vi "DAQmx devices info.vi"() -> (0 "ArrayInfo":string[][](array[string]))   [LabVIEW 2018]
doc: "Ricava, in <B>ArrayInfo</B>, informazioni sui dispositivi installati"
uses:
  <resource>/objmgr/daqmx.rc
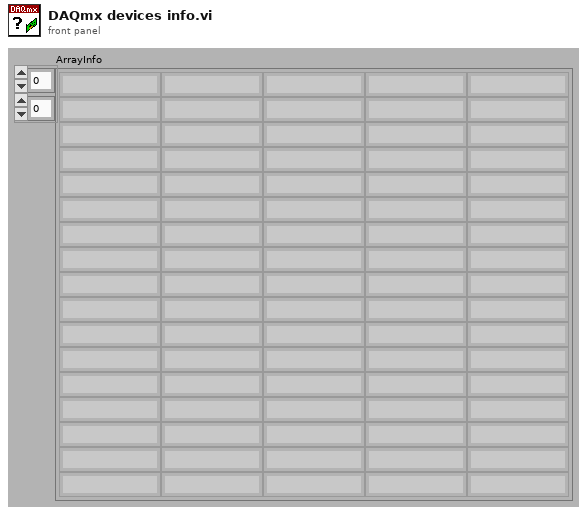
[diagram p1: front panel]
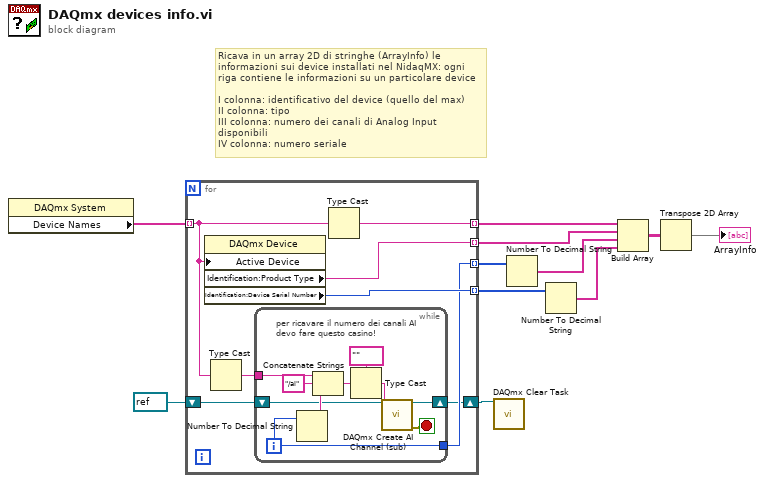
[diagram p0: block diagram]
diagram:
  # "Ricava in un array 2D di stringhe (ArrayInfo) le informazioni sui device installati nel NidaqMX: ogni riga contiene le informazioni su un particolare device\n\nI colonna: identificativo del device (quello del max)\nII colonna: tipo\nIII colonna: numero dei canali di Analog Input disponibili\nIV colonna: numero seriale"
  n1 = property class="DAQmx System"() -> ("Device Names"=w11:tag[])  [unwired: 2 in, 2 out]
  n2 = for {
    tunnel: w11 -> [w15] mode=indexing
    tunnel: [w19] -> w7 mode=indexing
    tunnel: [w18] -> w10 mode=indexing
    tunnel: [w16] -> w9 mode=indexing
    tunnel: [w14] -> w8 mode=indexing
    shift-right: [w13] -> w2
    shift-left: refnum<k21> refnum ("task in") -> [w12]
    n3 = property class="DAQmx Device"("Active Device"=w15) -> ("Identification:Product Type"=w19:string, "Identification:Device Serial Number"=w18:u32)  [unwired: 2 in, 2 out]
    n4 = Type Cast(x=w15) -> (*(type *) &x=w17:string)  [unwired: 1 in]
    n5 = while {
      tunnel: w17 -> [w28]
      tunnel: [w22] -> w16
      shift-right: [w20] -> w13
      shift-left: w12 -> [w24]
      i -> [w22]
      stop <- w21 stop-if-true
      # "per ricavare il numero dei canali AI devo fare questo casino!"
      n6 = Number To Decimal String(number=w22) -> (decimal integer string=w26:string)  [unwired: 1 in]
      n7 = Concatenate Strings(w28, "/ai" ("string"), w26) -> (w25:string)
      n8 = Type Cast(type=tag "", x=w25) -> (*(type *) &x=w23:tag)
      n9 = call <vilib>:"DAQmx Create AI Channel (sub).vi"("task in"=w24, "physical channel name"=w23) -> ("task out"=w20:refnum<k21>, "error out"=w21:errorcluster)  [unwired: 11 in, 1 out]
    }
    n10 = Type Cast(x=w15) -> (*(type *) &x=w14:string)  [unwired: 1 in]
  }
  n11 = call <vilib>:"DAQmx Clear Task.vi"("task in"=w2) -> ()  [unwired: 14 in, 1 out]
  n12 = Number To Decimal String(number=w9) -> (decimal integer string=w6:string[])  [unwired: 1 in]
  n13 = Number To Decimal String(number=w10) -> (decimal integer string=w5:string[])  [unwired: 1 in]
  n14 = Build Array(w8, w7, w6, w5) -> (w4:string[][])
  n15 = Transpose 2D Array(2D array=w4) -> (transposed array=→"ArrayInfo":string[][])
